vi "RotateXY.vi"(8 "Angle":dbl, 10 "Y":i16[](array[numeric]), 11 "X":i16[](array[numeric])) -> (2 "Yout":i16[](array[numeric]), 3 "Xout":i16[](array[numeric]))   [LabVIEW 2014]
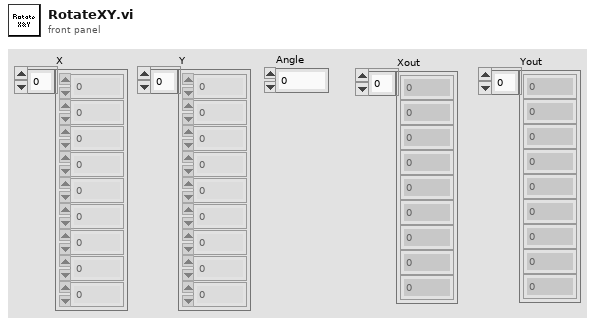
[diagram p1: front panel]
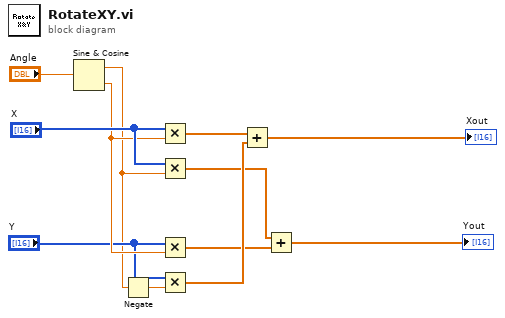
[diagram p0: block diagram]
diagram:
  n1 = Sine & Cosine(0:"Angle") -> (1:w7:dbl, 2:w10:dbl)
  n2 = Negate(x=w7) -> (-x=w8:dbl)
  n3 = Multiply(x="X", y=w10) -> (x*y=w6:dbl[])
  n4 = Multiply(x="X", y=w7) -> (x*y=w3:dbl[])
  n5 = Multiply(x="Y", y=w10) -> (x*y=w2:dbl[])
  n6 = Multiply(x="Y", y=w8) -> (x*y=w5:dbl[])
  n7 = Add(x=w6, y=w5) -> (x+y=→"Xout":dbl[])
  n8 = Add(x=w3, y=w2) -> (x+y=→"Yout":dbl[])
